vi "LoadImageInPictureBox.vi"(7 "Pict Refnum In":refnum<vi>, 8 "error in (no error)":errorcluster, 11 "Image file path":path) -> (0 "error out":errorcluster)   [LabVIEW 2011]
uses:
  <vilib>/picture/picture.llb/imagedata.ctl
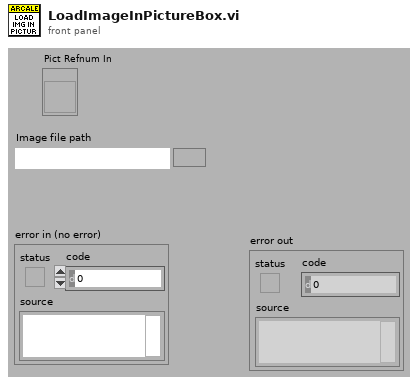
[diagram p1: front panel]
types:
  T1 = typedef "imagedata.ctl" = cluster{"image type":i32, "image depth":i32, "image":u8[], "mask":u8[], "colors":u32[], "Rectangle":cluster{"left":i16, "top":i16, "right":i16, "bottom":i16}}
  T2 = typedef "LVBoundsTypeDef.ctl" = cluster{"Width":u32, "Height":u32}
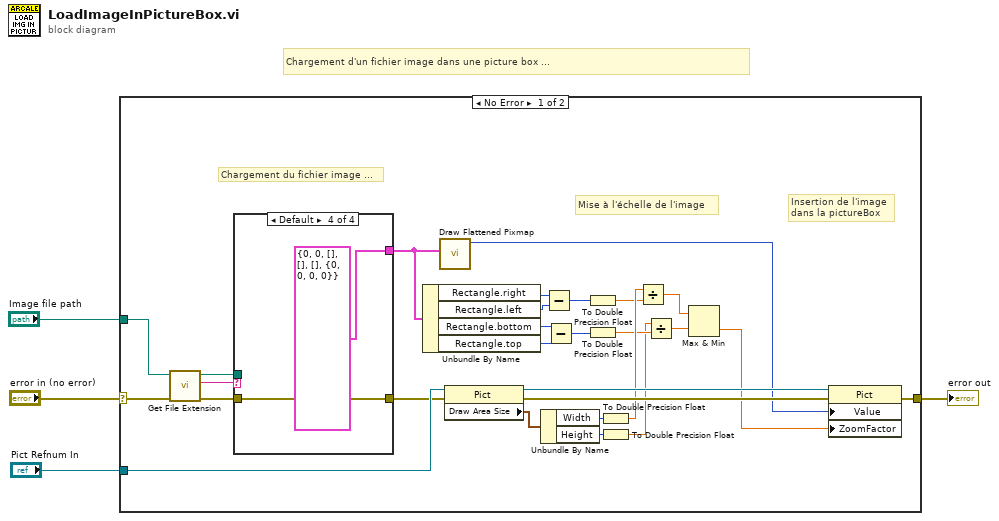
[diagram p0: block diagram]
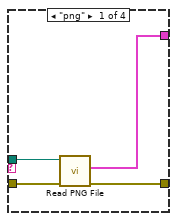
[diagram p2: hidden frame]
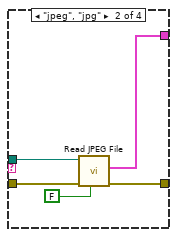
[diagram p3: hidden frame]
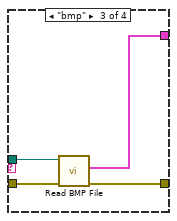
[diagram p4: hidden frame]
diagram:
  # "Chargement d'un fichier image dans une picture box ..."
  n1 = case shown="No Error" "error in (no error)" {
    selector: "error in (no error)" -> [w32 w48]
    tunnel: "Pict Refnum In" -> [w27 _]
    tunnel: [w26 w48] -> w3
    tunnel: "Image file path" -> [w31 _]
    frame No Error {
      # "Insertion de l'image\ndans la pictureBox"
      # "Mise à l'échelle de l'image"
      # "Chargement du fichier image ..."
      n2 = call <vilib>:"Get File Extension.vi"("error in (no error)"=w32, "file"=w31) -> ("error out"=w29:errorcluster, "lowercase file extension"=w30:string, "dup file"=w28:path)  [unwired: 6 in, 1 out]
      n3 = case shown="Default" w30 {
        tunnel: w29 -> [w36 w41 w45 w47]
        tunnel: w28 -> [w35 w39 w43 _]
        tunnel: [w33 w38 w42 T1 {"image type"=0, "image depth"=0, "image"=[], "mask"=[], "colors"=[], "Rectangle"={"left"=0, "top"=0, "right"=0, "bottom"=0}} ("image data")] -> w22
        tunnel: [w34 w37 w44 w47] -> w23
        frame "png" {
          n4 = call <vilib>:"Read PNG File.vi"("error in (no error)"=w36, "path to PNG file"=w35) -> ("error out"=w34:errorcluster, "image data"=w33:T1)  [unwired: 7 in, 1 out]
        }
        frame "jpeg", "jpg" {
          n5 = call <vilib>:"Read JPEG File.vi"("use 8 bit color table"=FALSE, "error in (no error)"=w41, "path to JPEG file"=w39) -> ("error out"=w37:errorcluster, "image data"=w38:T1)  [unwired: 6 in, 1 out]
        }
        frame "bmp" {
          n6 = call <vilib>:"Read BMP File.vi"("error in (no error)"=w45, "path to BMP file"=w43) -> ("error out"=w44:errorcluster, "image data"=w42:T1)  [unwired: 7 in, 1 out]
        }
        frame Default {
        }
      }
      n7 = Unbundle By Name(w22) -> ("Rectangle.right"=w21:i16, "Rectangle.left"=w20:i16, "Rectangle.bottom"=w19:i16, "Rectangle.top"=w18:i16)
      n8 = call <vilib>:"Draw Flattened Pixmap.vi"("image data"=w22) -> ("new picture"=w14:picture)  [unwired: 8 in]
      n9 = property class="Pict"(reference=w27, error in=w23) -> (reference out=w25:refnum<vi>, error out=w24:errorcluster, "Draw Area Size"=w17:T2)
      n10 = Unbundle By Name(w17) -> ("Width"=w16:u32, "Height"=w15:u32)
      n11 = Subtract(x=w21, y=w20) -> (x-y=w7:i16)
      n12 = Subtract(x=w19, y=w18) -> (x-y=w6:i16)
      n13 = To Double Precision Float(number=w7) -> (double precision float=w12:dbl)
      n14 = To Double Precision Float(number=w6) -> (double precision float=w11:dbl)
      n15 = To Double Precision Float(number=w16) -> (double precision float=w13:dbl)
      n16 = To Double Precision Float(number=w15) -> (double precision float=w10:dbl)
      n17 = Divide(x=w13, y=w12) -> (x/y=w8:dbl)
      n18 = Divide(x=w10, y=w11) -> (x/y=w9:dbl)
      n19 = Max & Min(x=w8, y=w9) -> (min(x,y)=w5:dbl)  [unwired: 1 out]
      n20 = property class="Pict"(reference=w25, error in=w24, "Value"=w14, "ZoomFactor"=w5) -> (error out=w26:errorcluster)  [unwired: 1 out]
    }
    frame Error {
    }
  }
  "error out" <- w3
